vi "Phase Set.vi"(6 "Update":bool=TRUE, 7 "Phase Cycle":dbl format="%#_13g", 8 "error in (no error)":errorcluster, 9 "node":i32, 10 "idxChannel":i32, 11 "hdwf":i32) -> (0 "error out":errorcluster, 1 "func_out":i32, 5 "Phase Out":dbl)   [LabVIEW 2024, in "AD2 DLL.lvlib"]
uses:
  AD2 DLL.lvlib
  <vilib>/Digilent/AD2 Toolkit/AD2.lvlib
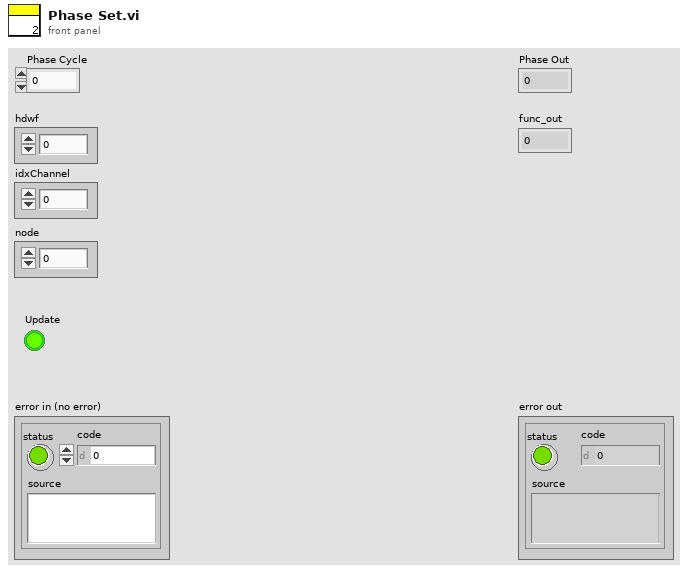
[diagram p1: front panel]
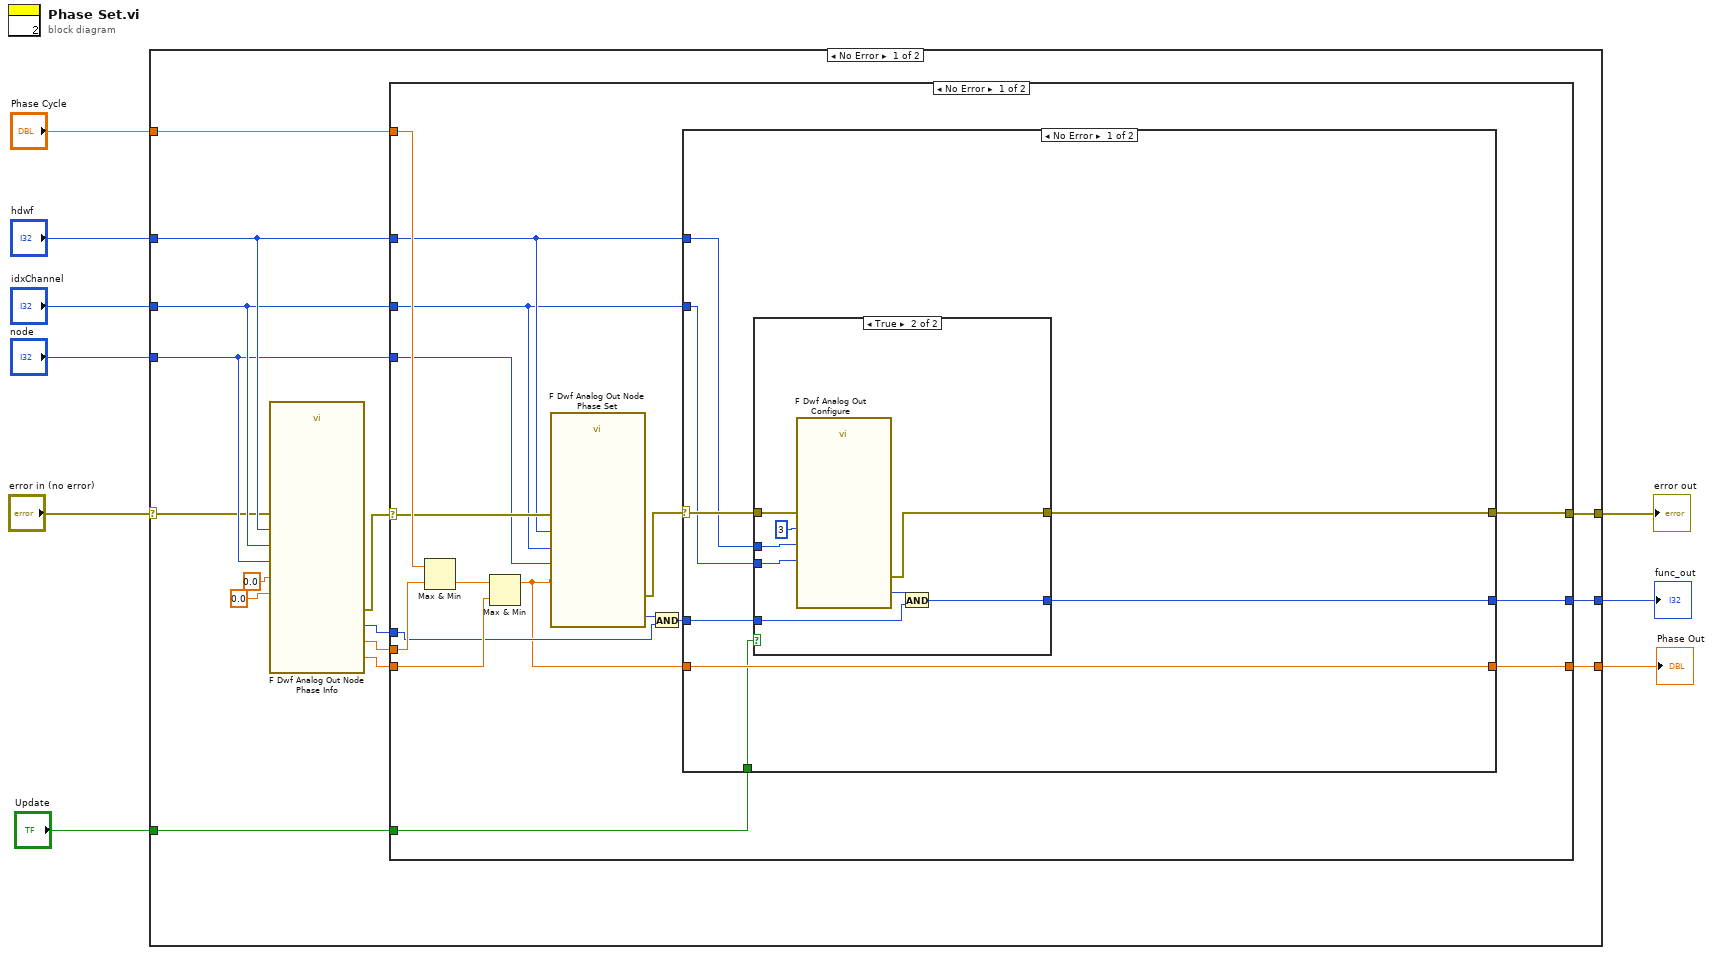
[diagram p0: block diagram]
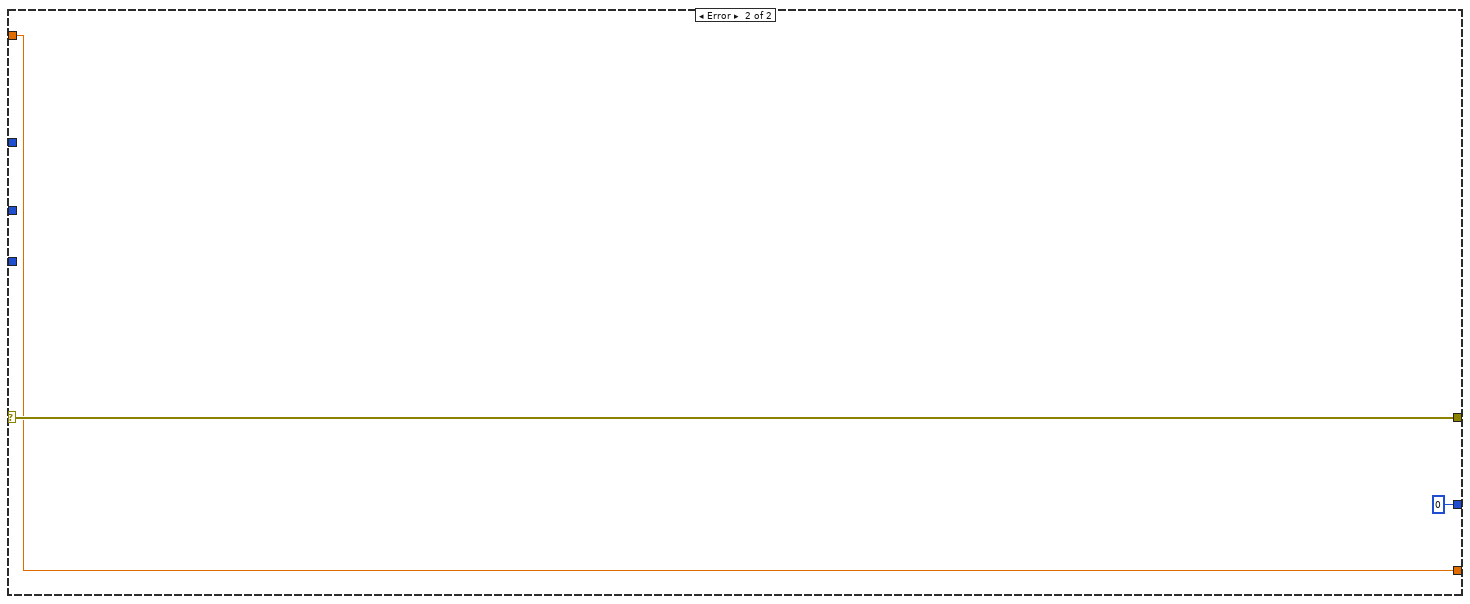
[diagram p5: hidden frame]
diagram:
  n1 = case shown="No Error" "error in (no error)" {
    selector: "error in (no error)" -> [w10 w68]
    tunnel: [w23 w68] -> w9
    tunnel: "hdwf" -> [w15 _]
    tunnel: "idxChannel" -> [w14 _]
    tunnel: "node" -> [w13 _]
    tunnel: "Phase Cycle" -> [w24 w66]
    tunnel: [w22 0] -> w3
    tunnel: [w21 w66] -> w2
    tunnel: "Update" -> [w20 _]
    frame No Error {
      n2 = call <vilib>:"F Dwf Analog Out Node Phase Info.vi"("pdegreeMax"=0.0, "pdegreeMin"=0.0, "error in (no error)"=w10, "node"=w13, "idxChannel"=w14, "hdwf"=w15) -> ("error out"=w19:errorcluster, "function return"=w18:i32, "pdegreeMax out"=w17:dbl, "pdegreeMin out"=w16:dbl)  [unwired: 2 in]
      n3 = case shown="No Error" w19 {
        selector: w19 -> [w28 w65]
        tunnel: w24 -> [w41 w63]
        tunnel: w17 -> [w40 _]
        tunnel: w16 -> [w38 _]
        tunnel: [w37 w65] -> w23
        tunnel: w15 -> [w27 _]
        tunnel: w14 -> [w26 _]
        tunnel: w13 -> [w25 _]
        tunnel: w18 -> [w36 w64]
        tunnel: [w34 w64] -> w22
        tunnel: [w33 w63] -> w21
        tunnel: w20 -> [w32 _]
        frame No Error {
          n4 = Max & Min(x=w41, y=w40) -> (min(x,y)=w39:dbl)  [unwired: 1 out]
          n5 = Max & Min(x=w39, y=w38) -> (max(x,y)=w29:dbl)  [unwired: 1 out]
          n6 = call <vilib>:"F Dwf Analog Out Node Phase Set.vi"("degreePhase"=w29, "error in (no error)"=w28, "node"=w25, "idxChannel"=w26, "hdwf"=w27) -> ("error out"=w31:errorcluster, "function return"=w30:i32)  [unwired: 5 in]
          n7 = And(x=w30, y=w36) -> (x .and. y?=w35:i32)
          n8 = case shown="No Error" w31 {
            selector: w31 -> [w49 w62]
            tunnel: [w46 w62] -> w37
            tunnel: w27 -> [w48 _]
            tunnel: w26 -> [w47 _]
            tunnel: w35 -> [w45 w61]
            tunnel: [w44 w61] -> w34
            tunnel: w29 -> [w43 w60]
            tunnel: [w43 w60] -> w33
            tunnel: w32 -> [w42 _]
            frame No Error {
              n9 = case shown="True" w42 {
                tunnel: w49 -> [w51 w59]
                tunnel: w48 -> [_ w57]
                tunnel: w47 -> [_ w56]
                tunnel: [w51 w55] -> w46
                tunnel: w45 -> [w50 w53]
                tunnel: [w50 w52] -> w44
                frame False {
                }
                frame True {
                  n10 = call <vilib>:"F Dwf Analog Out Configure.vi"("error in (no error)"=w59, "fStart"=3, "idxChannel"=w56, "hdwf"=w57) -> ("error out"=w55:errorcluster, "function return"=w54:i32)  [unwired: 6 in]
                  n11 = And(x=w54, y=w53) -> (x .and. y?=w52:i32)
                }
              }
            }
            frame Error {
            }
          }
        }
        frame Error {
        }
      }
    }
    frame Error {
    }
  }
  "error out" <- w9
  "func_out" <- w3
  "Phase Out" <- w2
